vi "executeCommand.vi"(8 "error in (no error)":errorcluster, 9 "input":variant, 10 "Command":T1=enum."getGratingWheelPosition", 11 "SpectrographClientCommunicator in":refnum<class "SpectrographClientCommunicator.lvclass">) -> (0 "error out":errorcluster, 2 "Output":string, 3 "SpectrographClientCommunicator out":refnum<class "SpectrographClientCommunicator.lvclass">)   [LabVIEW 2016, in "SpectrographClientCommunicator.lvclass"]
uses:
  SpectrographClientCommunicator.lvclass
  SpectrographTypeDef/SpectrographCMDs.ctl
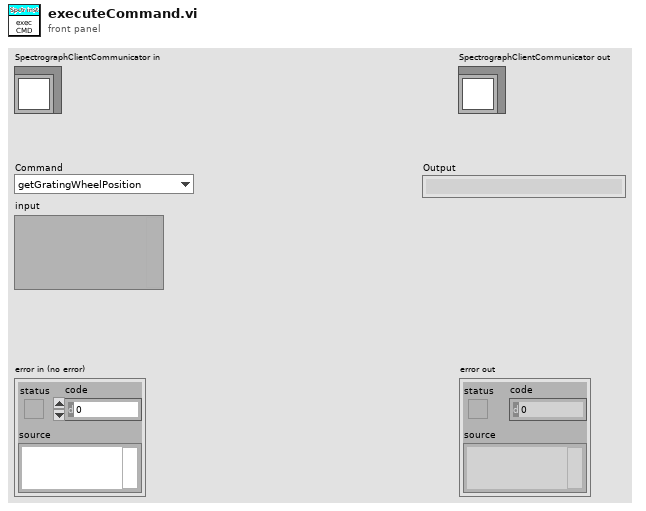
[diagram p1: front panel]
types:
  T1 = typedef "SpectrographCMDs.ctl" = enum16{"getFilterWheelPosition", "getGratingWheelPosition", "moveLinearStage", "moveGratingWheel", "moveFilterWheel", "homeLinearStage", "getLinearStageStatus", "getGratingWheelStatus", "getFilterWheelStatus", "stopAllMotion"}
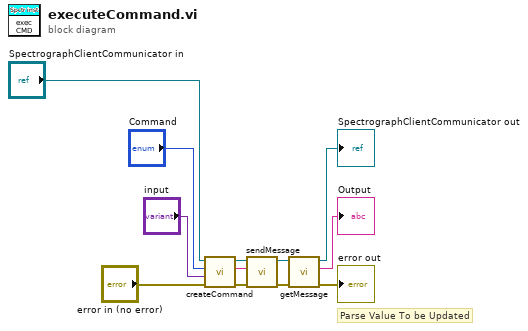
[diagram p0: block diagram]
diagram:
  # "Parse Value To be Updated"
  n1 = call "createCommand.vi"("error in (no error)"="error in (no error)", "Variant"="input", "Command"="Command", "SpectrographClientCommunicator in"="SpectrographClientCommunicator in") -> ("error out"=w8:errorcluster, "command"=w7:string, "SpectrographClientCommunicator out"=w6:refnum<class "SpectrographClientCommunicator.lvclass">)  [unwired: 5 in]
  n2 = call "sendMessage.vi"("error in (no error)"=w8, "message"=w7, "SpectrographClientCommunicator in"=w6) -> ("error out"=w4:errorcluster, "SpectrographClientCommunicator out"=w5:refnum<class "SpectrographClientCommunicator.lvclass">)  [unwired: 7 in]
  n3 = call "getMessage.vi"("error in (no error)"=w4, "SpectrographClientCommunicator in"=w5) -> ("error out"=→"error out":errorcluster, "message"=→"Output":string, "SpectrographClientCommunicator out"=→"SpectrographClientCommunicator out":refnum<class "SpectrographClientCommunicator.lvclass">)  [unwired: 7 in]
